vi "build_temp_array.vi"(1 "Array":fxp<+/-,24,5>[](array[numeric])=[0.0, 0.0, 0.0, 0.0, 0.0, 0.0, 0.0, 0.0, 0.0, 0.0, 0.0, 0.0, 0.0, 0.0, 0.0]) -> ()   [LabVIEW 2018]
uses:
  <vilib>/Platform/TimedLoop/XDataNode/timing_clust.ctl
  <vilib>/Platform/TimedLoop/XDataNode/nitl_modes.ctl
  <vilib>/Platform/TimedLoop/XDataNode/wakeup.ctl
  <vilib>/rvi/Emulation/niFpgaSctlEmulationGetInTimedLoop.vi
  <vilib>/rvi/Emulation/niFpgaEmulationReportErrorSimple.vi
  <vilib>/rvi/Emulation/niFpgaGetClockAttributes.vi
  <vilib>/rvi/Emulation/niFpgaCriticalErrorInLSC.vi
  <vilib>/Platform/TimedLoop/XDataNode/XDataNode.xnode
  <vilib>/Platform/TimedLoop/XDataNode/XDNodeRunTimeDep.lvlib
panel:
  out "fxp_T_extra1":i32
  out "fxp_T_pneum":i32
  out "fxp_T_pod":i32
  out "fxp_T_avb_r":i32
  out "fxp_T_avb_p2":i32
  out "fxp_T_avb_p1":i32
  out "fxp_T_piston7":i32
  out "fxp_T_piston6":i32
  out "fxp_T_piston5":i32
  out "fxp_T_extra2":i32
  out "fxp_T_piston4":i32
  out "fxp_T_piston3":i32
  out "fxp_T_piston2":i32
  out "fxp_T_piston1":i32
  out "fxp_T_piston0":i32
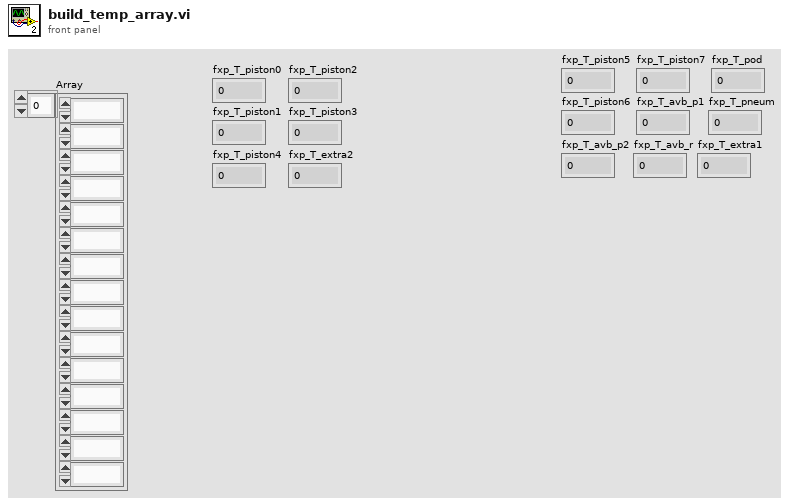
[diagram p1: front panel]
types:
  T1 = typedef "XDNodeRunTimeDep.lvlib/timing_clust.ctl" = cluster{"Expected End [f-1]":u64, "Actual End [f-1]":u64, "Finished Late? [f-1]":bool, "Expected End [i-1]":u64, "Actual End [i-1]":u64, "Finished Late? [i-1]":bool, "Expected Start [i]":u64, "Actual Start [i]":u64, "Expected Start [f]":u64, "Actual Start [f]":u64, "Source Name":string, "Structure Name":string, "Period":i64, "Deadline":i64, "Offset":i64, "Start":i64, "Priority":i32, "Timeout":i32, "Mode":T2, "Wakeup Reason":T3, "Error":errorcluster, "Source Type":string, "Secondary Source Type":string, "Global End Time":u64, "Global Start Time":u64, "Frame Duration":u64, "Iteration Duration":u64, "Assigned CPU":i32, "I/O Scan Engine Mode":u32}
  T2 = typedef "XDNodeRunTimeDep.lvlib/nitl_modes.ctl" = enum32{"No Change", "Process missed periods, maintain original phase", "Discard missed periods, maintain original phase", "Process missed periods, ignore original phase", "Discard missed periods, ignore original phase"}
  T3 = typedef "XDNodeRunTimeDep.lvlib/wakeup.ctl" = enum32{"Normal", "Aborted", "Asynchronous wakeup", "Timing source error", "Timed loop error", "Timeout"}
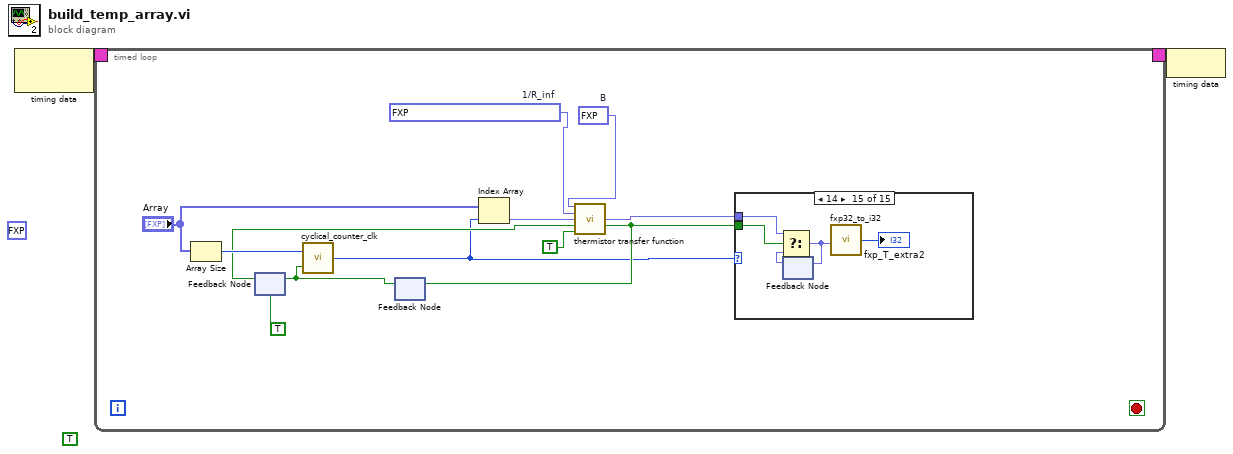
[diagram p0: block diagram]
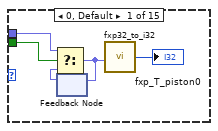
[diagram p2: hidden frame]
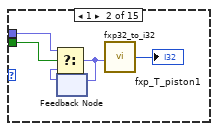
[diagram p3: hidden frame]
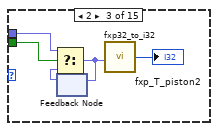
[diagram p4: hidden frame]
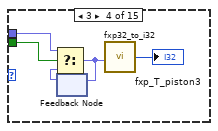
[diagram p5: hidden frame]
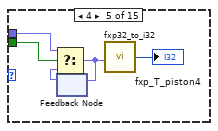
[diagram p6: hidden frame]
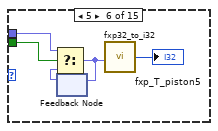
[diagram p7: hidden frame]
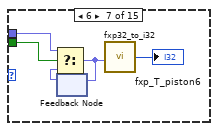
[diagram p8: hidden frame]
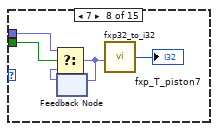
[diagram p9: hidden frame]
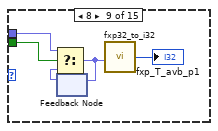
[diagram p10: hidden frame]
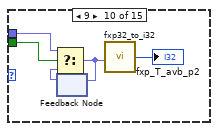
[diagram p11: hidden frame]
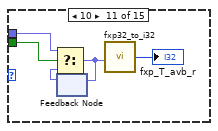
[diagram p12: hidden frame]
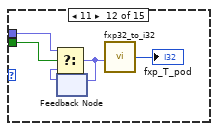
[diagram p13: hidden frame]
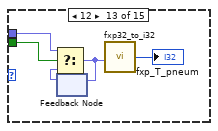
[diagram p14: hidden frame]
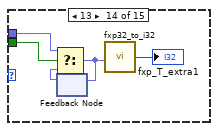
[diagram p15: hidden frame]
diagram:
  (unwired) TRUE
  (unwired) fxp<+,2,2> 0.0
  n1 = node-c288() -> (w2:T1)  [unwired: 1 in]
  n2 = timed-loop {
    timing: w2 -> [_]
    timing-out: [_] -> w1
    stop <- _ stop-if-true
    w11 = fxp<+,32,7> 10.047783523797989  # 1/R_inf
    w12 = fxp<+/-,32,16> 3434.0  # B
    n3 = Array Size(array="Array") -> (size(s)=w9:i32)
    n4 = feedback #1(TRUE ("ready for input")) -> (w6:bool)
    n5 = feedback #2() -> (w4:bool)  [unwired: 1 in]
    n6 = feedback-in #1(w4) -> ()
    n7 = call "cyclical_counter_clk.vi"("clk"=w4, "Mod"=w9) -> ("Count"=w3:u16)
    n8 = Index Array(array="Array", index=w3) -> (element=w13:fxp<+/-,24,5>)
    n9 = call "thermistor transfer function.vi"("B"=w12, "1/R_inf"=w11, "V"=w13, "input valid"=w6, "ready for output (T)"=TRUE) -> ("Temperature"=w10:fxp<+/-,32,16>, "output valid"=w5:bool)  [unwired: 8 in, 1 out]
    n10 = feedback-in #2(w5) -> ()
    n11 = case shown="14" w3 {
      tunnel: w5 -> [w16 w21 w26 w31 w36 w41 w46 w51 w56 w61 w66 w71 w76 w81 w86]
      tunnel: w10 -> [w19 w24 w29 w34 w39 w44 w49 w54 w59 w64 w69 w74 w79 w84 w89]
      frame 0, Default {
        n12 = feedback #3() -> (w17:fxp<+/-,32,16>)  [unwired: 1 in]
        n13 = Select(t=w19, s=w16, f=w17) -> (s? t:f=w18:fxp<+/-,32,16>)
        n14 = feedback-in #3(w18) -> ()
        n15 = call "fxp32_to_i32.vi"("fxp32_16"=w18) -> ("32bit integer"=→"fxp_T_piston0":i32)
      }
      frame 1 {
        n16 = feedback #4() -> (w22:fxp<+/-,32,16>)  [unwired: 1 in]
        n17 = Select(t=w24, s=w21, f=w22) -> (s? t:f=w23:fxp<+/-,32,16>)
        n18 = feedback-in #4(w23) -> ()
        n19 = call "fxp32_to_i32.vi"("fxp32_16"=w23) -> ("32bit integer"=→"fxp_T_piston1":i32)
      }
      frame 2 {
        n20 = feedback #5() -> (w27:fxp<+/-,32,16>)  [unwired: 1 in]
        n21 = Select(t=w29, s=w26, f=w27) -> (s? t:f=w28:fxp<+/-,32,16>)
        n22 = feedback-in #5(w28) -> ()
        n23 = call "fxp32_to_i32.vi"("fxp32_16"=w28) -> ("32bit integer"=→"fxp_T_piston2":i32)
      }
      frame 3 {
        n24 = feedback #6() -> (w32:fxp<+/-,32,16>)  [unwired: 1 in]
        n25 = Select(t=w34, s=w31, f=w32) -> (s? t:f=w33:fxp<+/-,32,16>)
        n26 = feedback-in #6(w33) -> ()
        n27 = call "fxp32_to_i32.vi"("fxp32_16"=w33) -> ("32bit integer"=→"fxp_T_piston3":i32)
      }
      frame 4 {
        n28 = feedback #7() -> (w37:fxp<+/-,32,16>)  [unwired: 1 in]
        n29 = Select(t=w39, s=w36, f=w37) -> (s? t:f=w38:fxp<+/-,32,16>)
        n30 = feedback-in #7(w38) -> ()
        n31 = call "fxp32_to_i32.vi"("fxp32_16"=w38) -> ("32bit integer"=→"fxp_T_piston4":i32)
      }
      frame 5 {
        n32 = feedback #8() -> (w42:fxp<+/-,32,16>)  [unwired: 1 in]
        n33 = Select(t=w44, s=w41, f=w42) -> (s? t:f=w43:fxp<+/-,32,16>)
        n34 = feedback-in #8(w43) -> ()
        n35 = call "fxp32_to_i32.vi"("fxp32_16"=w43) -> ("32bit integer"=→"fxp_T_piston5":i32)
      }
      frame 6 {
        n36 = feedback #9() -> (w47:fxp<+/-,32,16>)  [unwired: 1 in]
        n37 = Select(t=w49, s=w46, f=w47) -> (s? t:f=w48:fxp<+/-,32,16>)
        n38 = feedback-in #9(w48) -> ()
        n39 = call "fxp32_to_i32.vi"("fxp32_16"=w48) -> ("32bit integer"=→"fxp_T_piston6":i32)
      }
      frame 7 {
        n40 = feedback #10() -> (w52:fxp<+/-,32,16>)  [unwired: 1 in]
        n41 = Select(t=w54, s=w51, f=w52) -> (s? t:f=w53:fxp<+/-,32,16>)
        n42 = feedback-in #10(w53) -> ()
        n43 = call "fxp32_to_i32.vi"("fxp32_16"=w53) -> ("32bit integer"=→"fxp_T_piston7":i32)
      }
      frame 8 {
        n44 = feedback #11() -> (w57:fxp<+/-,32,16>)  [unwired: 1 in]
        n45 = Select(t=w59, s=w56, f=w57) -> (s? t:f=w58:fxp<+/-,32,16>)
        n46 = feedback-in #11(w58) -> ()
        n47 = call "fxp32_to_i32.vi"("fxp32_16"=w58) -> ("32bit integer"=→"fxp_T_avb_p1":i32)
      }
      frame 9 {
        n48 = feedback #12() -> (w62:fxp<+/-,32,16>)  [unwired: 1 in]
        n49 = Select(t=w64, s=w61, f=w62) -> (s? t:f=w63:fxp<+/-,32,16>)
        n50 = feedback-in #12(w63) -> ()
        n51 = call "fxp32_to_i32.vi"("fxp32_16"=w63) -> ("32bit integer"=→"fxp_T_avb_p2":i32)
      }
      frame 10 {
        n52 = feedback #13() -> (w67:fxp<+/-,32,16>)  [unwired: 1 in]
        n53 = Select(t=w69, s=w66, f=w67) -> (s? t:f=w68:fxp<+/-,32,16>)
        n54 = feedback-in #13(w68) -> ()
        n55 = call "fxp32_to_i32.vi"("fxp32_16"=w68) -> ("32bit integer"=→"fxp_T_avb_r":i32)
      }
      frame 11 {
        n56 = feedback #14() -> (w72:fxp<+/-,32,16>)  [unwired: 1 in]
        n57 = Select(t=w74, s=w71, f=w72) -> (s? t:f=w73:fxp<+/-,32,16>)
        n58 = feedback-in #14(w73) -> ()
        n59 = call "fxp32_to_i32.vi"("fxp32_16"=w73) -> ("32bit integer"=→"fxp_T_pod":i32)
      }
      frame 12 {
        n60 = feedback #15() -> (w77:fxp<+/-,32,16>)  [unwired: 1 in]
        n61 = Select(t=w79, s=w76, f=w77) -> (s? t:f=w78:fxp<+/-,32,16>)
        n62 = feedback-in #15(w78) -> ()
        n63 = call "fxp32_to_i32.vi"("fxp32_16"=w78) -> ("32bit integer"=→"fxp_T_pneum":i32)
      }
      frame 13 {
        n64 = feedback #16() -> (w82:fxp<+/-,32,16>)  [unwired: 1 in]
        n65 = Select(t=w84, s=w81, f=w82) -> (s? t:f=w83:fxp<+/-,32,16>)
        n66 = feedback-in #16(w83) -> ()
        n67 = call "fxp32_to_i32.vi"("fxp32_16"=w83) -> ("32bit integer"=→"fxp_T_extra1":i32)
      }
      frame 14 {
        n68 = feedback #17() -> (w87:fxp<+/-,32,16>)  [unwired: 1 in]
        n69 = Select(t=w89, s=w86, f=w87) -> (s? t:f=w88:fxp<+/-,32,16>)
        n70 = feedback-in #17(w88) -> ()
        n71 = call "fxp32_to_i32.vi"("fxp32_16"=w88) -> ("32bit integer"=→"fxp_T_extra2":i32)
      }
    }
  }
  n72 = node-c288(w1) -> ()
